vi "List Symbols.vi"(8 "error in (no error)":errorcluster, 11 "AMS Connection In":T1) -> (0 "Error Out":errorcluster, 3 "Symbols":T3[](array[typedef]) {"dataType" format="%x" items=["INT"=2, "BOOL"=33]; "iOffs" format="%.0x"; "iGroup" format="%.0x"; "entryLength" format="%.0x"})   [LabVIEW 2017, in "TwinCAT ADS.lvlib" / "PLC.lvlib"]
doc: "Returns a list of available <b>Symbols</b> on the target device."
uses:
  PLC.lvlib
  TypeDefs/AdsSymbolEntry.ctl
  TypeDefs/dataType.ctl
  Low Level/TypeDefs/AMS Connection.ctl
  Low Level/TypeDefs/AMS.ctl
  TwinCAT ADS.lvlib
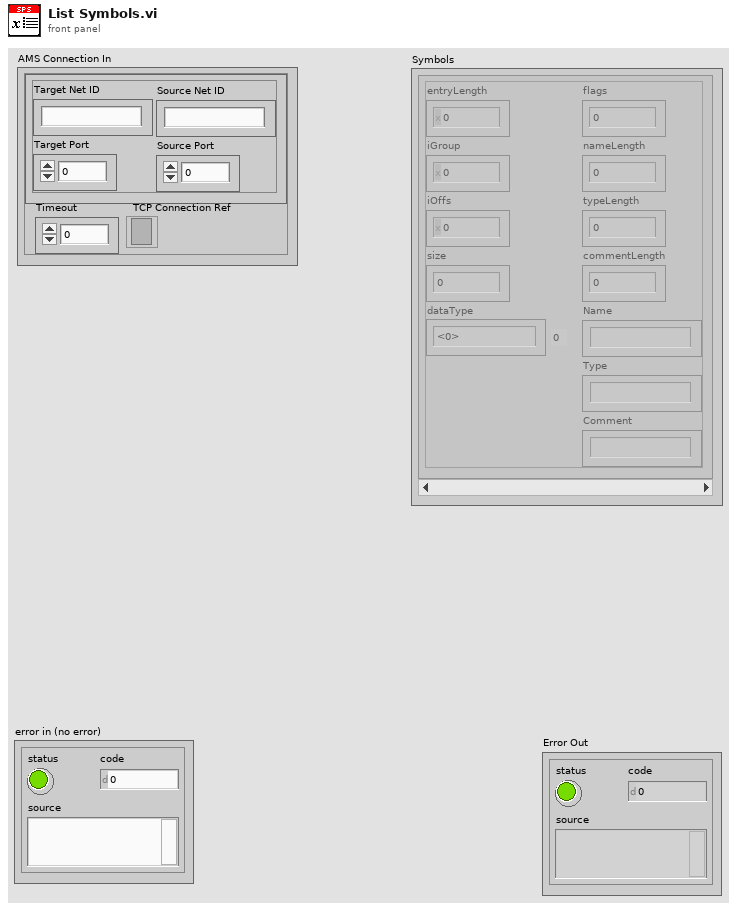
[diagram p1: front panel]
types:
  T1 = typedef "TwinCAT ADS.lvlib/AMS Connection.ctl" = cluster{"AMS":T2, "Timeout":i32, "TCP Connection Ref":refnum<k5>}
  T2 = typedef "TwinCAT ADS.lvlib/AMS.ctl" = cluster{"Target Net ID":string, "Target Port":u16, "Source Net ID":string, "Source Port":u16}
  T3 = typedef "TwinCAT ADS.lvlib/PLC.lvlib/AdsSymbolEntry.ctl" = cluster{"entryLength":i32, "iGroup":i32, "iOffs":i32, "size":i32, "dataType":T4, "flags":i32, "nameLength":i16, "typeLength":i16, "commentLength":i16, "Name":string, "Type":string, "Comment":string}
  T4 = typedef "TwinCAT ADS.lvlib/PLC.lvlib/dataType.ctl" = u16
  T5 = typedef "TwinCAT ADS.lvlib/ADS Error.ctl" = i32
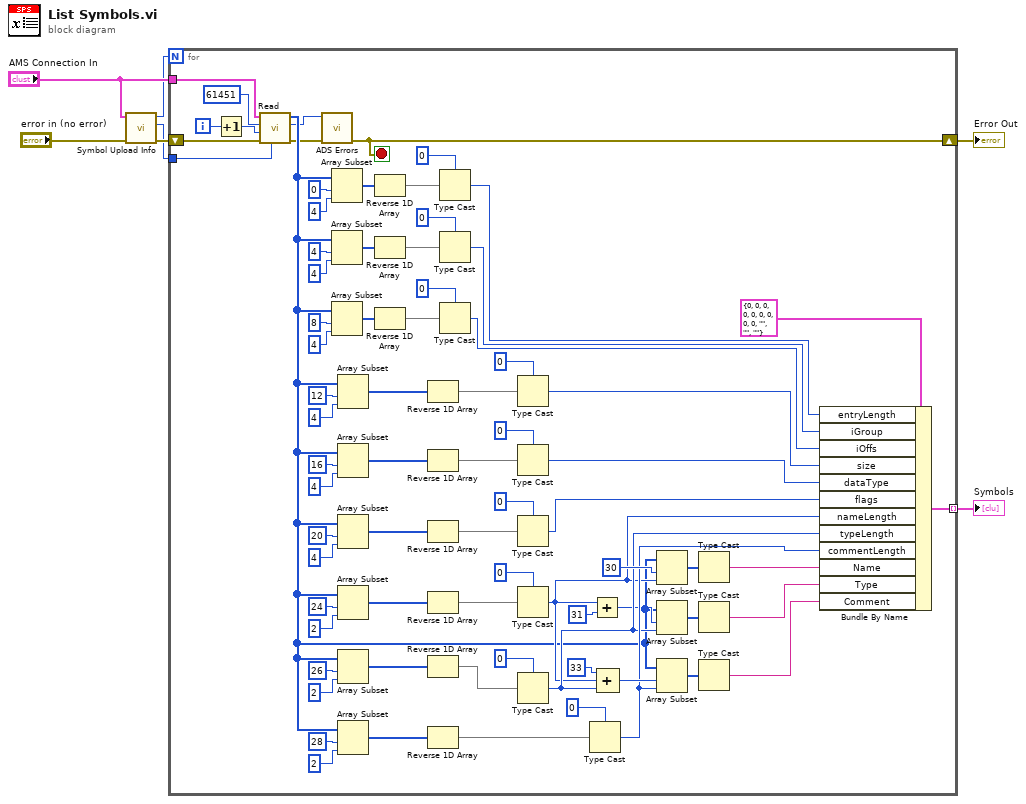
[diagram p0: block diagram]
diagram:
  n1 = call "Symbol Upload Info.vi"("Error In"="error in (no error)", "AMS Connection In"="AMS Connection In") -> ("Error Out"=w6:errorcluster, "Symsize"=w1:u32, "Symbols"=w2:u32)  [unwired: 7 in]
  n2 = for {
    N: w2 -> [_]
    tunnel: [w63] -> w7 mode=indexing
    tunnel: w1 -> [w62]
    shift-right: [w8] -> w4
    shift-left: w6 -> [w61]
    tunnel: "AMS Connection In" -> [w13]
    i -> [w83]
    stop <- w8 stop-if-true
    n3 = Increment(x=w83) -> (x+1=w11:i32)
    n4 = call "Read.vi"("Read Length"=w62, "Error In"=w61, "Offset"=w11, "Index Group"=u32 61451, "AMS Connection In"=w13) -> ("Error Out"=w10:errorcluster, "ADS Error"=w9:T5, "Data"=w12:u8[])  [unwired: 4 in]
    n5 = call "ADS Errors.vi"("error in (no error)"=w10, "ADS Error"=w9) -> ("error out"=w8:errorcluster)  [unwired: 9 in]
    n6 = Array Subset(array=w12, index=0, length=4) -> (w79:u8[])
    n7 = Array Subset(array=w12, index=4, length=4) -> (w73:u8[])
    n8 = Array Subset(array=w12, index=8, length=4) -> (w67:u8[])
    n9 = Array Subset(array=w12, index=12, length=4) -> (w58:u8[])
    n10 = Array Subset(array=w12, index=16, length=4) -> (w52:u8[])
    n11 = Array Subset(array=w12, index=20, length=4) -> (w48:u8[])
    n12 = Array Subset(array=w12, index=24, length=2) -> (w41:u8[])
    n13 = Array Subset(array=w12, index=26, length=2) -> (w38:u8[])
    n14 = Array Subset(array=w12, index=28, length=2) -> (w34:u8[])
    n15 = Reverse 1D Array(array=w79) -> (reversed array=w78:u8[])
    n16 = Reverse 1D Array(array=w73) -> (reversed array=w74:u8[])
    n17 = Reverse 1D Array(array=w67) -> (reversed array=w66:u8[])
    n18 = Reverse 1D Array(array=w58) -> (reversed array=w59:u8[])
    n19 = Reverse 1D Array(array=w52) -> (reversed array=w51:u8[])
    n20 = Reverse 1D Array(array=w48) -> (reversed array=w49:u8[])
    n21 = Reverse 1D Array(array=w41) -> (reversed array=w40:u8[])
    n22 = Reverse 1D Array(array=w38) -> (reversed array=w39:u8[])
    n23 = Reverse 1D Array(array=w34) -> (reversed array=w33:u8[])
    n24 = Type Cast(type=0 ("Read Length"), x=w78) -> (*(type *) &x=w77:i32)
    n25 = Type Cast(type=0 ("Read Length"), x=w74) -> (*(type *) &x=w70:i32)
    n26 = Type Cast(type=0 ("Read Length"), x=w66) -> (*(type *) &x=w64:i32)
    n27 = Type Cast(type=0 ("Read Length"), x=w59) -> (*(type *) &x=w55:i32)
    n28 = Type Cast(type=0 ("Read Length"), x=w51) -> (*(type *) &x=w50:i32)
    n29 = Type Cast(type=0 ("Read Length"), x=w49) -> (*(type *) &x=w24:i32)
    n30 = Type Cast(type=i16 0 ("Read Length"), x=w40) -> (*(type *) &x=w16:i16)
    n31 = Type Cast(type=i16 0 ("Read Length"), x=w39) -> (*(type *) &x=w18:i16)
    n32 = Type Cast(type=i16 0 ("Read Length"), x=w33) -> (*(type *) &x=w23:i16)
    n33 = Add(x=w16, y=31 ("index")) -> (x+y=w17:i32)
    n34 = Compound Arithmetic op=unknown(33 ("index"), w16, w18) -> (w25:i32)
    n35 = Array Subset(array=w12, index=30, length=w16) -> (w28:u8[])
    n36 = Array Subset(array=w12, index=w17, length=w18) -> (w15:u8[])
    n37 = Array Subset(array=w12, index=w25, length=w23) -> (w22:u8[])
    n38 = Type Cast(x=w28) -> (*(type *) &x=w27:string)  [unwired: 1 in]
    n39 = Type Cast(x=w15) -> (*(type *) &x=w20:string)  [unwired: 1 in]
    n40 = Type Cast(x=w22) -> (*(type *) &x=w21:string)  [unwired: 1 in]
    n41 = Bundle By Name(cluster=T3 {"entryLength"=0, "iGroup"=0, "iOffs"=0, "size"=0, "dataType"=0, "flags"=0, "nameLength"=0, "typeLength"=0, "commentLength"=0, "Name"="", "Type"="", "Comment"=""} ("AdsSymbolEntry"), "entryLength"=w77, "iGroup"=w70, "iOffs"=w64, "size"=w55, "dataType"=w50, "flags"=w24, "nameLength"=w16, "typeLength"=w18, "commentLength"=w23, "Name"=w27, "Type"=w20, "Comment"=w21) -> (w63:T3)
  }
  "Symbols" <- w7
  "Error Out" <- w4
